vi "Matrix (2D) to Array (1D).vi"(4 "Matrix (2D)":T1) -> (1 "Array (1D)":dbl[](array[numeric]))   [LabVIEW 2014]
uses:
  <vilib>/Analysis/Matrix/Datatypes/RealMatrix.ctl
  <vilib>/Analysis/Matrix/NI_Matrix.lvlib
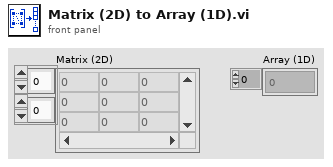
[diagram p1: front panel]
types:
  T1 = typedef "NI_Matrix.lvlib/RealMatrix.ctl" = dbl[][]
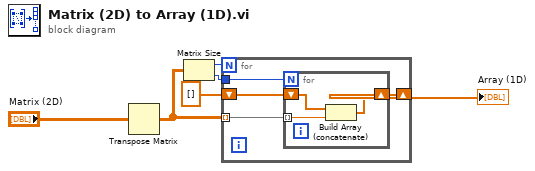
[diagram p0: block diagram]
diagram:
  n1 = Transpose Matrix(1:"Matrix (2D)") -> (0:w2:T1)
  n2 = Matrix Size(0:w2) -> (1:w3:i32, 2:w4:i32)
  n3 = for {
    N: w3 -> [_]
    tunnel: w2 -> [w9] mode=indexing
    tunnel: w4 -> [w8]
    shift-right: [w10] -> w5
    shift-left: dbl[] [] -> [w7]
    n4 = for {
      N: w8 -> [_]
      tunnel: w9 -> [w13] mode=indexing
      shift-right: [w12] -> w10
      shift-left: w7 -> [w11]
      n5 = Build Array (concatenate)(w11, w13) -> (w12:dbl[])
    }
  }
  "Array (1D)" <- w5
